vi "Find Controllers.vi"(8 "Error In":errorcluster) -> (0 "Error Out":errorcluster, 3 "Xbox Controllers":T1[](array[typedef]))   [LabVIEW 2021, in "LMH-Xbox-One-Controller.lvlib"]
doc: "Find all Xbox controllers and return device index."
uses:
  <instrlib>/Xbox-One-Controller/LMH-Xbox-One-Controller.lvlib
  <instrlib>/Xbox-One-Controller/Private/Type Defs/Xbox Controller Device.ctl
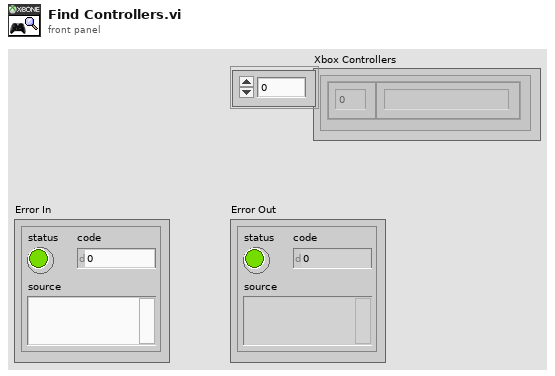
[diagram p1: front panel]
types:
  T1 = typedef "LMH-Xbox-One-Controller.lvlib/Xbox Controller Device.ctl" = cluster{"Device Index":i32, "Device Name":string}
  T2 = cluster{"axes total":u32, "buttons total":u32, "pov total":u32, "device name":string}[]
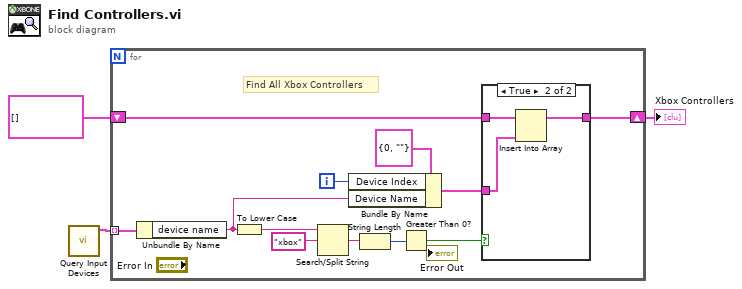
[diagram p0: block diagram]
diagram:
  n1 = call <vilib>:"Query Input Devices.vi"() -> ("joystick info"=w3:T2)  [unwired: 8 in, 3 out]
  n2 = for {
    tunnel: w3 -> [w15] mode=indexing
    shift-right: [w4] -> w1
    shift-left: T1[] [] -> [w5]
    i -> [w9]
    # "Find All Xbox Controllers"
    n3 = Unbundle By Name(w15) -> ("device name"=w8:string)
    n4 = To Lower Case(string=w8) -> (all lower case string=w14:string)
    n5 = Search/Split String(string=w14, search string/char (-)="xbox") -> (match + rest of string=w12:string)  [unwired: 1 in, 2 out]
    n6 = Bundle By Name(cluster=T1 {"Device Index"=0, "Device Name"=""} ("Xbox Controllers"), "Device Index"=w9, "Device Name"=w8) -> (w6:T1)
    n7 = String Length(string=w12) -> (length=w11:i32)
    n8 = Greater Than 0?(x=w11) -> (x > 0?=w7:bool)
    n9 = case shown="True" w7 {
      tunnel: w6 -> [_ w17]
      tunnel: w5 -> [w16 w19]
      tunnel: [w16 w18] -> w4
      frame False {
      }
      frame True {
        n10 = Insert Into Array(array=w19, new element=w17) -> (w18:T1[])  [unwired: 1 in]
      }
    }
  }
  "Xbox Controllers" <- w1
